vi "持续时间&充气时间.vi"() -> (0 "气密保持压力持续时间":string, 2 "气密充气时间":string)   [LabVIEW 2015]
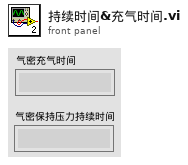
[diagram p1: front panel]
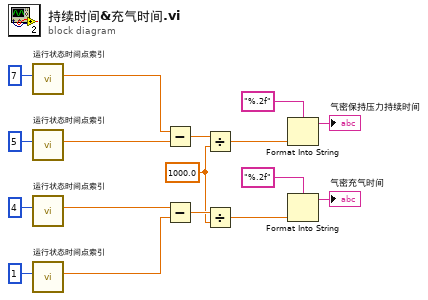
[diagram p0: block diagram]
diagram:
  w15 = 1000.0 ("y")
  n1 = call "运行状态时间点索引.vi"("索引"=7) -> ("数值"=w3:dbl)  [unwired: 10 in]
  n2 = call "运行状态时间点索引.vi"("索引"=5) -> ("数值"=w4:dbl)  [unwired: 10 in]
  n3 = call "运行状态时间点索引.vi"("索引"=4) -> ("数值"=w9:dbl)  [unwired: 10 in]
  n4 = call "运行状态时间点索引.vi"("索引"=1) -> ("数值"=w7:dbl)  [unwired: 10 in]
  n5 = Subtract(x=w3, y=w4) -> (x-y=w16:dbl)
  n6 = Subtract(x=w9, y=w7) -> (x-y=w17:dbl)
  n7 = Divide(x=w16, y=w15) -> (x/y=w12:dbl)
  n8 = Divide(x=w17, y=w15) -> (x/y=w14:dbl)
  n9 = Format Into String(format string="%.2f" ("格式字符串"), w12) -> (resulting string=→"气密保持压力持续时间":string)  [unwired: 2 in, 1 out]
  n10 = Format Into String(format string="%.2f" ("格式字符串"), w14) -> (resulting string=→"气密充气时间":string)  [unwired: 2 in, 1 out]
